vi "复检判定.vi"(7 "Result":refnum<vi>, 10 "判定参数":T1, 11 "XY曲线":cluster{"X":dbl[], "Y":dbl[]}[](array[cluster])) -> (3 "OK？":bool)   [LabVIEW 2020]
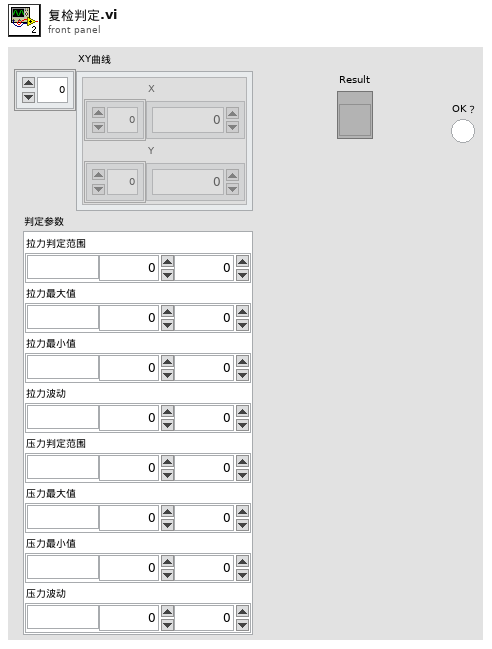
[diagram p1: front panel]
types:
  T1 = cluster{"拉力判定范围":cluster{"单位":string, "下限":dbl, "上限":dbl}, "拉力最大值":cluster{"单位":string, "下限":dbl, "上限":dbl}, "拉力最小值":cluster{"单位":string, "下限":dbl, "上限":dbl}, "拉力波动":cluster{"单位":string, "下限":dbl, "上限":dbl}, "压力判定范围":cluster{"单位":string, "下限":dbl, "上限":dbl}, "压力最大值":cluster{"单位":string, "下限":dbl, "上限":dbl}, "压力最小值":cluster{"单位":string, "下限":dbl, "上限":dbl}, "压力波动":cluster{"单位":string, "下限":dbl, "上限":dbl}}
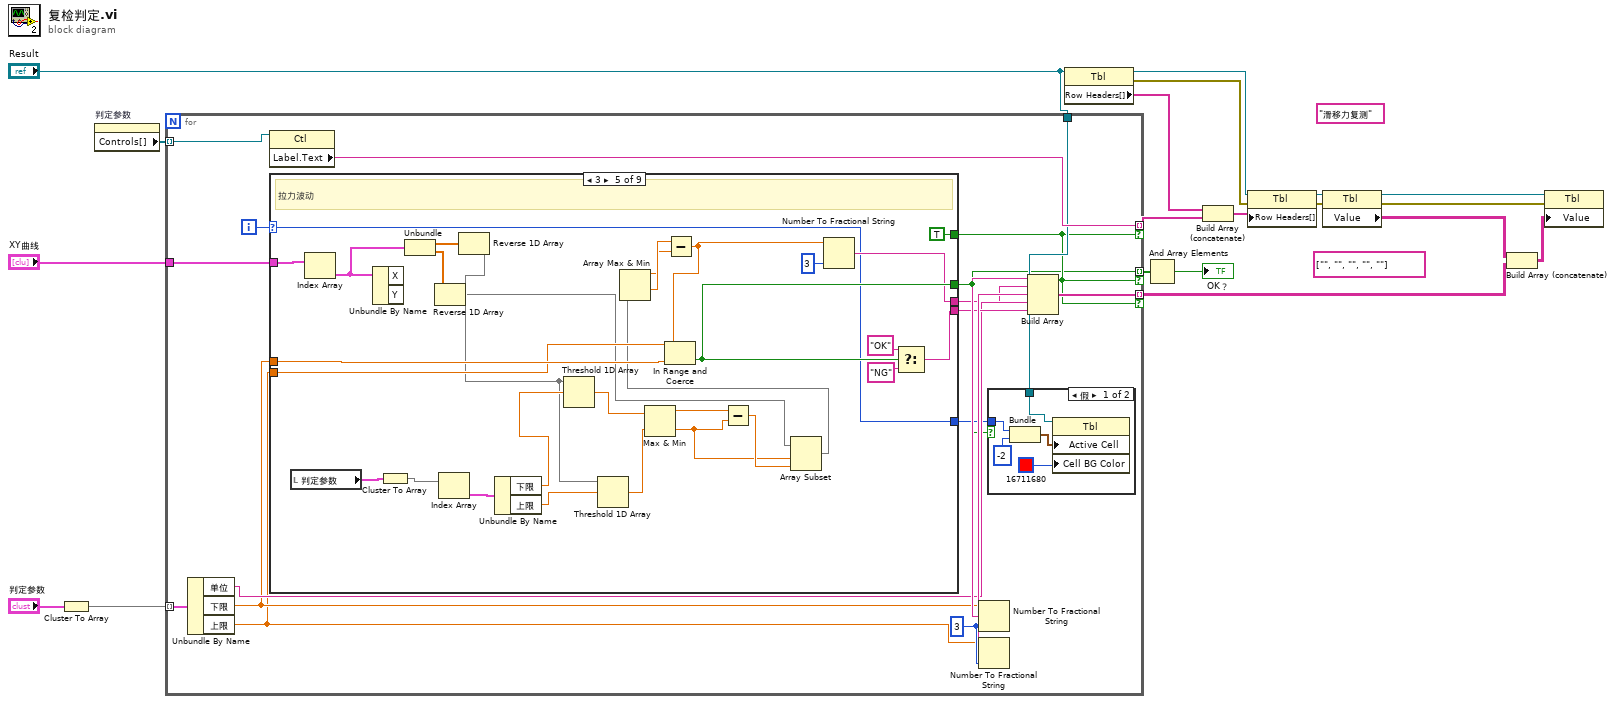
[diagram p0: block diagram]
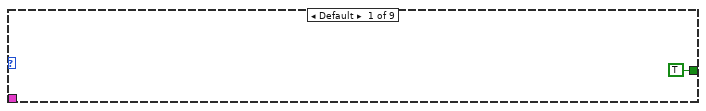
[diagram p3: hidden frame]
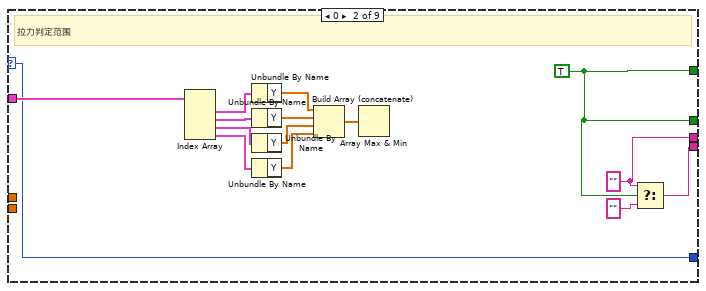
[diagram p4: hidden frame]
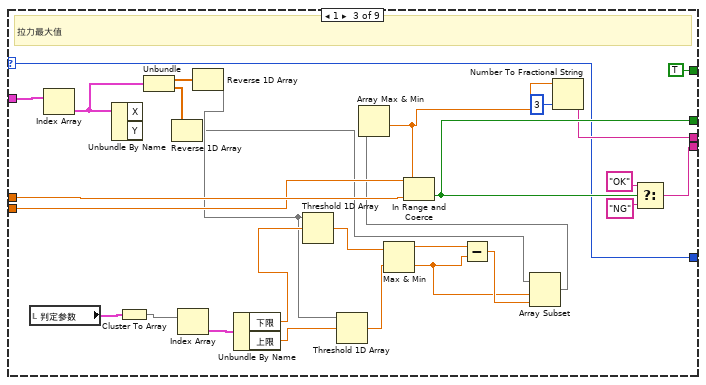
[diagram p5: hidden frame]
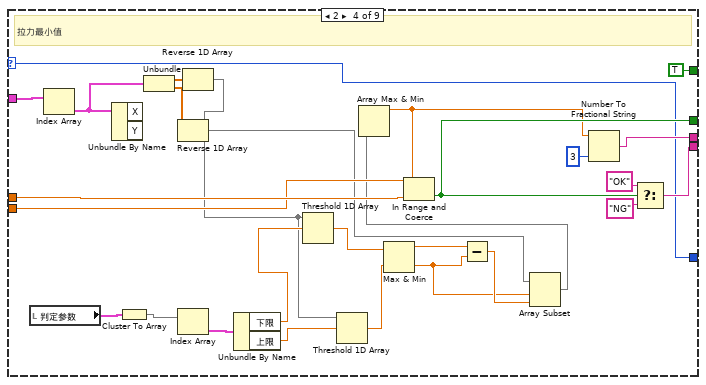
[diagram p6: hidden frame]
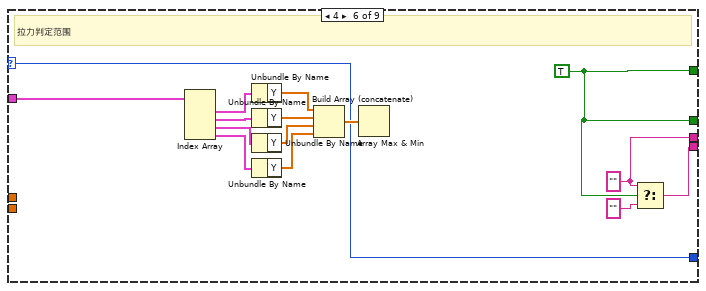
[diagram p7: hidden frame]
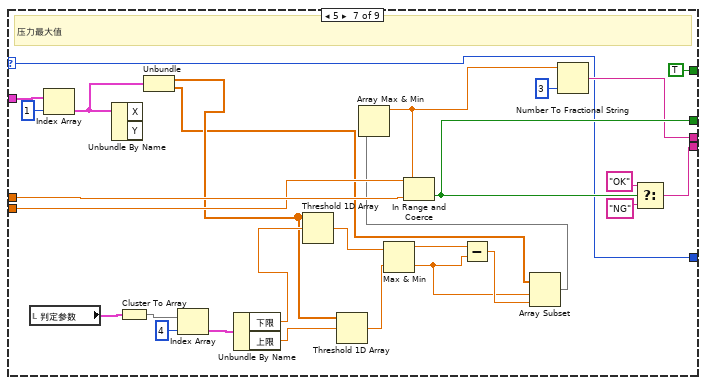
[diagram p8: hidden frame]
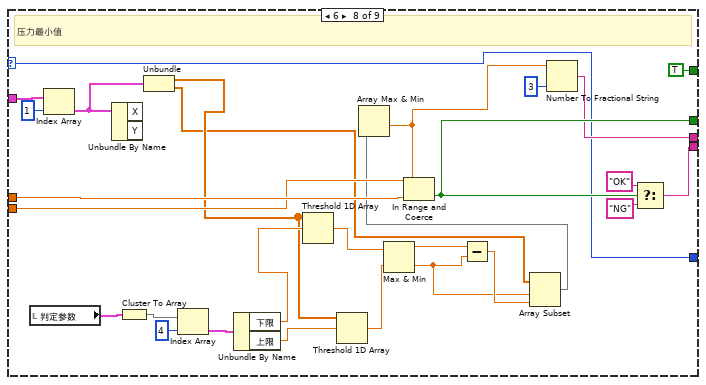
[diagram p9: hidden frame]
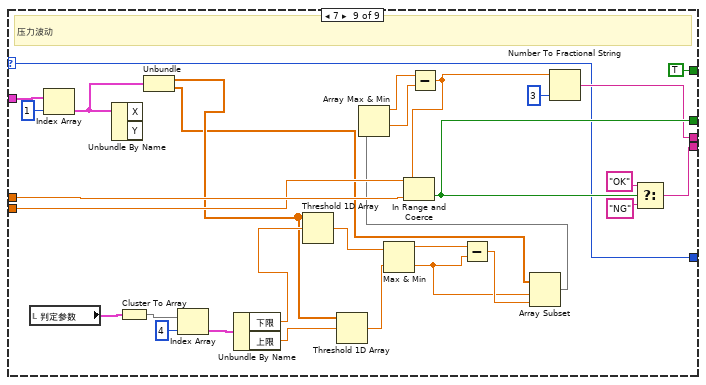
[diagram p10: hidden frame]
diagram:
  (unwired) string[] ["", "", "", "", ""]
  (unwired) "滑移力复测" ("Label.Text")
  n1 = Cluster To Array(cluster="判定参数") -> (array=w19:cluster{"单位":string, "下限":dbl, "上限":dbl}[])
  n2 = property on="判定参数" class="Clust (严格)"() -> ("Controls[]"=w17:refnum<vi>[])  [unwired: 2 in, 2 out]
  n3 = for {
    tunnel: w19 -> [w37] mode=indexing
    tunnel: w17 -> [w35] mode=indexing
    tunnel: "XY曲线" -> [w34]
    tunnel: [w20] -> w15 mode=indexing if=w22
    tunnel: [w26] -> w2 mode=indexing if=w22
    tunnel: [w25] -> w4 mode=indexing if=w22
    tunnel: "Result" -> [w23]
    i -> [w36]
    w33 = i16 3 ("精度(6)")
    n4 = Unbundle By Name(w37) -> ("单位"=w29:string, "下限"=w28:dbl, "上限"=w27:dbl)
    n5 = property class="Ctl"(reference=w35) -> ("Label.Text"=w25:string)  [unwired: 1 in, 2 out]
    n6 = case shown="3" w36 {
      selector: w36 -> [_ w44 w61 w89 w117 w145 w160 w188 w216]
      tunnel: w34 -> [_ w58 w86 w114 w144 w159 w187 w215 w245]
      tunnel: [_ w47 w83 w111 w141 w148 w184 w212 w242] -> w30
      tunnel: [_ w46 w82 w110 w140 w147 w183 w211 w241] -> w20
      tunnel: w28 -> [_ _ w81 w109 w139 _ w182 w210 w240]
      tunnel: w27 -> [_ _ w80 w108 w138 _ w181 w209 w239]
      tunnel: [TRUE w46 TRUE TRUE TRUE w147 TRUE TRUE TRUE] -> w22
      tunnel: [_ w45 w62 w91 w118 w146 w161 w189 w217] -> w24
      tunnel: [_ w44 w61 w89 w117 w145 w160 w188 w216] -> w21
      frame Default {
      }
      frame 0 {
        w46 = TRUE
        w45 = ""
        # "拉力判定范围"
        n7 = Index Array(array=w58) -> (element #1=w57:cluster{"X":dbl[], "Y":dbl[]}, element #2=w54:cluster{"X":dbl[], "Y":dbl[]}, element #3=w55:cluster{"X":dbl[], "Y":dbl[]}, element #4=w56:cluster{"X":dbl[], "Y":dbl[]})  [unwired: 4 in]
        n8 = Unbundle By Name(w57) -> ("Y"=w53:dbl[])
        n9 = Unbundle By Name(w54) -> ("Y"=w52:dbl[])
        n10 = Unbundle By Name(w55) -> ("Y"=w51:dbl[])
        n11 = Unbundle By Name(w56) -> ("Y"=w50:dbl[])
        n12 = Build Array (concatenate)(w53, w52, w51, w50) -> (w49:dbl[])
        n13 = Array Max & Min(array=w49) -> ()  [unwired: 4 out]
        n14 = Select(t=w45, s=w46, f="") -> (s? t:f=w47:string)
      }
      frame 1 {
        # "拉力最大值"
        n15 = local read "判定参数"() -> (w78:T1)
        n16 = Index Array(array=w86) -> (element=w70:cluster{"X":dbl[], "Y":dbl[]})  [unwired: 1 in]
        n17 = Unbundle By Name(w70) -> ()  [unwired: 2 out]
        n18 = Cluster To Array(cluster=w78) -> (array=w77:cluster{"单位":string, "下限":dbl, "上限":dbl}[])
        n19 = Unbundle(w70) -> ("X"=w69:dbl[], "Y"=w66:dbl[])
        n20 = Reverse 1D Array(array=w66) -> (reversed array=w59:dbl[])
        n21 = Index Array(array=w77) -> (element=w76:cluster{"单位":string, "下限":dbl, "上限":dbl})  [unwired: 1 in]
        n22 = Reverse 1D Array(array=w69) -> (reversed array=w60:dbl[])
        n23 = Unbundle By Name(w76) -> ("下限"=w75:dbl, "上限"=w73:dbl)
        n24 = Threshold 1D Array(2:w75, 3:w60) -> (0:w74:dbl)  [unwired: 1 in]
        n25 = Threshold 1D Array(2:w73, 3:w60) -> (0:w72:dbl)  [unwired: 1 in]
        n26 = Max & Min(x=w74, y=w72) -> (max(x,y)=w71:dbl, min(x,y)=w67:dbl)
        n27 = Subtract(x=w71, y=w67) -> (x-y=w68:dbl)
        n28 = Array Subset(array=w59, index=w67, length=w68) -> (w65:dbl[])
        n29 = Array Max & Min(array=w65) -> (min value=w64:dbl)  [unwired: 3 out]
        n30 = In Range and Coerce(upper limit=w80, x=w64, lower limit=w81) -> (In Range?=w82:bool)  [unwired: 1 out]
        n31 = Number To Fractional String(number=w64, precision (6)=i16 3 ("精度(6)")) -> (F-format string=w62:string)  [unwired: 2 in]
        n32 = Select(t="OK", s=w82, f="NG") -> (s? t:f=w83:string)
      }
      frame 2 {
        # "拉力最小值"
        n33 = local read "判定参数"() -> (w106:T1)
        n34 = Index Array(array=w114) -> (element=w98:cluster{"X":dbl[], "Y":dbl[]})  [unwired: 1 in]
        n35 = Unbundle By Name(w98) -> ()  [unwired: 2 out]
        n36 = Cluster To Array(cluster=w106) -> (array=w105:cluster{"单位":string, "下限":dbl, "上限":dbl}[])
        n37 = Unbundle(w98) -> ("X"=w97:dbl[], "Y"=w94:dbl[])
        n38 = Reverse 1D Array(array=w94) -> (reversed array=w87:dbl[])
        n39 = Index Array(array=w105) -> (element=w104:cluster{"单位":string, "下限":dbl, "上限":dbl})  [unwired: 1 in]
        n40 = Reverse 1D Array(array=w97) -> (reversed array=w88:dbl[])
        n41 = Unbundle By Name(w104) -> ("下限"=w103:dbl, "上限"=w101:dbl)
        n42 = Threshold 1D Array(2:w103, 3:w88) -> (0:w102:dbl)  [unwired: 1 in]
        n43 = Threshold 1D Array(2:w101, 3:w88) -> (0:w100:dbl)  [unwired: 1 in]
        n44 = Max & Min(x=w102, y=w100) -> (max(x,y)=w99:dbl, min(x,y)=w95:dbl)
        n45 = Subtract(x=w99, y=w95) -> (x-y=w96:dbl)
        n46 = Array Subset(array=w87, index=w95, length=w96) -> (w93:dbl[])
        n47 = Array Max & Min(array=w93) -> (max value=w90:dbl)  [unwired: 3 out]
        n48 = In Range and Coerce(upper limit=w108, x=w90, lower limit=w109) -> (In Range?=w110:bool)  [unwired: 1 out]
        n49 = Number To Fractional String(number=w90, precision (6)=i16 3 ("精度(6)")) -> (F-format string=w91:string)  [unwired: 2 in]
        n50 = Select(t="OK", s=w110, f="NG") -> (s? t:f=w111:string)
      }
      frame 3 {
        # "拉力波动"
        n51 = local read "判定参数"() -> (w136:T1)
        n52 = Index Array(array=w144) -> (element=w128:cluster{"X":dbl[], "Y":dbl[]})  [unwired: 1 in]
        n53 = Unbundle By Name(w128) -> ()  [unwired: 2 out]
        n54 = Cluster To Array(cluster=w136) -> (array=w135:cluster{"单位":string, "下限":dbl, "上限":dbl}[])
        n55 = Unbundle(w128) -> ("X"=w127:dbl[], "Y"=w124:dbl[])
        n56 = Reverse 1D Array(array=w124) -> (reversed array=w115:dbl[])
        n57 = Index Array(array=w135) -> (element=w134:cluster{"单位":string, "下限":dbl, "上限":dbl})  [unwired: 1 in]
        n58 = Reverse 1D Array(array=w127) -> (reversed array=w116:dbl[])
        n59 = Unbundle By Name(w134) -> ("下限"=w133:dbl, "上限"=w131:dbl)
        n60 = Threshold 1D Array(2:w133, 3:w116) -> (0:w132:dbl)  [unwired: 1 in]
        n61 = Threshold 1D Array(2:w131, 3:w116) -> (0:w130:dbl)  [unwired: 1 in]
        n62 = Max & Min(x=w132, y=w130) -> (max(x,y)=w129:dbl, min(x,y)=w125:dbl)
        n63 = Subtract(x=w129, y=w125) -> (x-y=w126:dbl)
        n64 = Array Subset(array=w115, index=w125, length=w126) -> (w123:dbl[])
        n65 = Array Max & Min(array=w123) -> (max value=w121:dbl, min value=w122:dbl)  [unwired: 2 out]
        n66 = Subtract(x=w122, y=w121) -> (x-y=w119:dbl)
        n67 = In Range and Coerce(upper limit=w138, x=w119, lower limit=w139) -> (In Range?=w140:bool)  [unwired: 1 out]
        n68 = Number To Fractional String(number=w119, precision (6)=i16 3 ("精度(6)")) -> (F-format string=w118:string)  [unwired: 2 in]
        n69 = Select(t="OK", s=w140, f="NG") -> (s? t:f=w141:string)
      }
      frame 4 {
        w147 = TRUE
        w146 = ""
        # "拉力判定范围"
        n70 = Index Array(array=w159) -> (element #1=w158:cluster{"X":dbl[], "Y":dbl[]}, element #2=w155:cluster{"X":dbl[], "Y":dbl[]}, element #3=w156:cluster{"X":dbl[], "Y":dbl[]}, element #4=w157:cluster{"X":dbl[], "Y":dbl[]})  [unwired: 4 in]
        n71 = Unbundle By Name(w158) -> ("Y"=w154:dbl[])
        n72 = Unbundle By Name(w155) -> ("Y"=w153:dbl[])
        n73 = Unbundle By Name(w156) -> ("Y"=w152:dbl[])
        n74 = Unbundle By Name(w157) -> ("Y"=w151:dbl[])
        n75 = Build Array (concatenate)(w154, w153, w152, w151) -> (w150:dbl[])
        n76 = Array Max & Min(array=w150) -> ()  [unwired: 4 out]
        n77 = Select(t=w146, s=w147, f="") -> (s? t:f=w148:string)
      }
      frame 5 {
        # "压力最大值"
        n78 = local read "判定参数"() -> (w179:T1)
        n79 = Index Array(array=w187, index=1 ("索引")) -> (element=w171:cluster{"X":dbl[], "Y":dbl[]})
        n80 = Unbundle By Name(w171) -> ()  [unwired: 2 out]
        n81 = Cluster To Array(cluster=w179) -> (array=w178:cluster{"单位":string, "下限":dbl, "上限":dbl}[])
        n82 = Unbundle(w171) -> ("X"=w170:dbl[], "Y"=w167:dbl[])
        n83 = Index Array(array=w178, index=4 ("索引")) -> (element=w177:cluster{"单位":string, "下限":dbl, "上限":dbl})
        n84 = Unbundle By Name(w177) -> ("下限"=w176:dbl, "上限"=w174:dbl)
        n85 = Threshold 1D Array(2:w176, 3:w170) -> (0:w175:dbl)  [unwired: 1 in]
        n86 = Threshold 1D Array(2:w174, 3:w170) -> (0:w173:dbl)  [unwired: 1 in]
        n87 = Max & Min(x=w175, y=w173) -> (max(x,y)=w172:dbl, min(x,y)=w168:dbl)
        n88 = Subtract(x=w172, y=w168) -> (x-y=w169:dbl)
        n89 = Array Subset(array=w167, index=w168, length=w169) -> (w166:dbl[])
        n90 = Array Max & Min(array=w166) -> (max value=w162:dbl)  [unwired: 3 out]
        n91 = In Range and Coerce(upper limit=w181, x=w162, lower limit=w182) -> (In Range?=w183:bool)  [unwired: 1 out]
        n92 = Number To Fractional String(number=w162, precision (6)=i16 3 ("精度(6)")) -> (F-format string=w161:string)  [unwired: 2 in]
        n93 = Select(t="OK", s=w183, f="NG") -> (s? t:f=w184:string)
      }
      frame 6 {
        # "压力最小值"
        n94 = local read "判定参数"() -> (w207:T1)
        n95 = Index Array(array=w215, index=1 ("索引")) -> (element=w199:cluster{"X":dbl[], "Y":dbl[]})
        n96 = Unbundle By Name(w199) -> ()  [unwired: 2 out]
        n97 = Cluster To Array(cluster=w207) -> (array=w206:cluster{"单位":string, "下限":dbl, "上限":dbl}[])
        n98 = Unbundle(w199) -> ("X"=w198:dbl[], "Y"=w195:dbl[])
        n99 = Index Array(array=w206, index=4 ("索引")) -> (element=w205:cluster{"单位":string, "下限":dbl, "上限":dbl})
        n100 = Unbundle By Name(w205) -> ("下限"=w204:dbl, "上限"=w202:dbl)
        n101 = Threshold 1D Array(2:w204, 3:w198) -> (0:w203:dbl)  [unwired: 1 in]
        n102 = Threshold 1D Array(2:w202, 3:w198) -> (0:w201:dbl)  [unwired: 1 in]
        n103 = Max & Min(x=w203, y=w201) -> (max(x,y)=w200:dbl, min(x,y)=w196:dbl)
        n104 = Subtract(x=w200, y=w196) -> (x-y=w197:dbl)
        n105 = Array Subset(array=w195, index=w196, length=w197) -> (w194:dbl[])
        n106 = Array Max & Min(array=w194) -> (min value=w190:dbl)  [unwired: 3 out]
        n107 = In Range and Coerce(upper limit=w209, x=w190, lower limit=w210) -> (In Range?=w211:bool)  [unwired: 1 out]
        n108 = Number To Fractional String(number=w190, precision (6)=i16 3 ("精度(6)")) -> (F-format string=w189:string)  [unwired: 2 in]
        n109 = Select(t="OK", s=w211, f="NG") -> (s? t:f=w212:string)
      }
      frame 7 {
        # "压力波动"
        n110 = local read "判定参数"() -> (w237:T1)
        n111 = Index Array(array=w245, index=1 ("索引")) -> (element=w229:cluster{"X":dbl[], "Y":dbl[]})
        n112 = Unbundle By Name(w229) -> ()  [unwired: 2 out]
        n113 = Cluster To Array(cluster=w237) -> (array=w236:cluster{"单位":string, "下限":dbl, "上限":dbl}[])
        n114 = Unbundle(w229) -> ("X"=w228:dbl[], "Y"=w225:dbl[])
        n115 = Index Array(array=w236, index=4 ("索引")) -> (element=w235:cluster{"单位":string, "下限":dbl, "上限":dbl})
        n116 = Unbundle By Name(w235) -> ("下限"=w234:dbl, "上限"=w232:dbl)
        n117 = Threshold 1D Array(2:w234, 3:w228) -> (0:w233:dbl)  [unwired: 1 in]
        n118 = Threshold 1D Array(2:w232, 3:w228) -> (0:w231:dbl)  [unwired: 1 in]
        n119 = Max & Min(x=w233, y=w231) -> (max(x,y)=w230:dbl, min(x,y)=w226:dbl)
        n120 = Subtract(x=w230, y=w226) -> (x-y=w227:dbl)
        n121 = Array Subset(array=w225, index=w226, length=w227) -> (w224:dbl[])
        n122 = Array Max & Min(array=w224) -> (max value=w221:dbl, min value=w220:dbl)  [unwired: 2 out]
        n123 = Subtract(x=w221, y=w220) -> (x-y=w218:dbl)
        n124 = In Range and Coerce(upper limit=w239, x=w218, lower limit=w240) -> (In Range?=w241:bool)  [unwired: 1 out]
        n125 = Number To Fractional String(number=w218, precision (6)=i16 3 ("精度(6)")) -> (F-format string=w217:string)  [unwired: 2 in]
        n126 = Select(t="OK", s=w241, f="NG") -> (s? t:f=w242:string)
      }
    }
    n127 = Number To Fractional String(number=w28, precision (6)=w33) -> (F-format string=w32:string)  [unwired: 2 in]
    n128 = Number To Fractional String(number=w27, precision (6)=w33) -> (F-format string=w31:string)  [unwired: 2 in]
    n129 = case shown="假" w20 {
      tunnel: w23 -> [w42 _]
      tunnel: w21 -> [w38 _]
      frame False {
        n130 = Bundle(w38, -2) -> (w40:cluster{i32, i32})  [unwired: 1 in]
        n131 = property class="Tbl"(reference=w42, "Active Cell"=w40, "Cell BG Color"=u32 16711680 ("活动单元格:单元格背景色")) -> ()  [unwired: 1 in, 2 out]
      }
      frame True {
      }
    }
    n132 = Build Array(w32, w24, w31, w29, w30) -> (w26:string[])
  }
  n133 = property class="Tbl"(reference="Result") -> (reference out=w6:refnum<vi>, error out=w11:errorcluster, "Row Headers[]"=w3:string[])  [unwired: 1 in]
  n134 = And Array Elements(Boolean array=w15) -> (logical AND=→"OK？":bool)
  n135 = Build Array (concatenate)(w3, w4) -> (w5:string[])
  n136 = property class="Tbl"(reference=w6, error in=w11, "Row Headers[]"=w5) -> (reference out=w7:refnum<vi>, error out=w10:errorcluster)
  n137 = property class="Tbl"(reference=w7, error in=w10) -> (reference out=w8:refnum<vi>, error out=w9:errorcluster, "Value"=w12:string[][])
  n138 = Build Array (concatenate)(w12, w2) -> (w13:string[][])
  n139 = property class="Tbl"(reference=w8, error in=w9, "Value"=w13) -> ()  [unwired: 2 out]
